vi "Initialise.vi"(8 "error in (no error)":errorcluster, 11 "Node in":refnum<class "bt_Send_Notifier.lvclass">) -> (0 "error out":errorcluster, 3 "Node out":refnum<class "bt_Send_Notifier.lvclass">)   [LabVIEW 2021, in "BT.lvlib" / "bt_Send_Notifier.lvclass"]
uses:
  bt_Send_Notifier.lvclass
  bt_Send_Notifier.lvclass/bt_Send_Notifier.ctl
  Properties/Read Name.vi
  With Values/Send/bt_Send_Synch_WithValues.lvclass
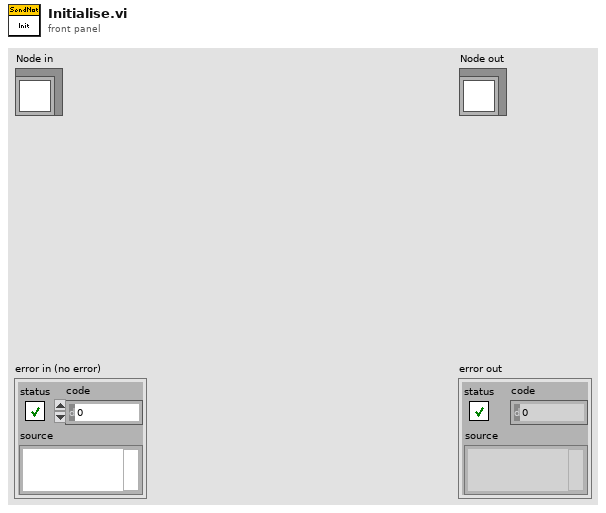
[diagram p1: front panel]
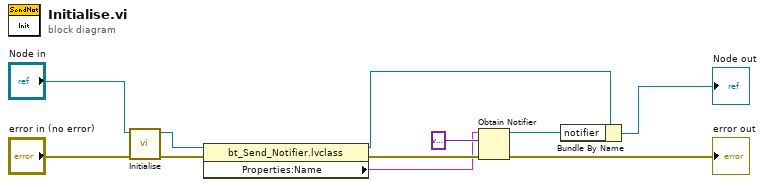
[diagram p0: block diagram]
diagram:
  n1 = call-parent "Initialise.vi"("error in (no error)"="error in (no error)", "Node in"="Node in") -> ("error out"=w6:errorcluster, "Node out"=w5:refnum<class "bt_Send_Notifier.lvclass">)  [unwired: 8 in]
  n2 = property class="bt_Send_Notifier.lvclass"(reference=w5, error in=w6) -> (reference out=w4:refnum<class "bt_Send_Notifier.lvclass">, error out=w3:errorcluster, "Properties:Name"=w2:string)
  n3 = Obtain Notifier(name (unnamed)=w2, notification data type=variant, error in (no error)=w3) -> (notifier out=w1:refnum<notifier>, error out=→"error out":errorcluster)  [unwired: 1 in, 1 out]
  n4 = Bundle By Name(cluster=w4, "notifier"=w1) -> (→"Node out":refnum<class "bt_Send_Notifier.lvclass">)
